vi "Teguh_2.vi"() -> ()   [LabVIEW 2024]
uses:
  <vilib>/Utility/NIReport.llb/Report Type.ctl
  <vilib>/MakerHub/LINX/Private/Device/Type Defs/Stimulus Pulse.ctl
  <vilib>/MakerHub/LINX/Public/Peripherals/Digital/Digital Write 1 Chan.vi
  <vilib>/MakerHub/LINX/Public/Peripherals/Digital/Digital Write N Chans.vi
  <vilib>/MakerHub/LINX/Private/Local IO/LinxDigitalWrite.vi
  <vilib>/MakerHub/LINX/Public/Utilities/Check Channel.vi
  <vilib>/MakerHub/LINX/Public/Utilities/Open Serial.vi
  <vilib>/MakerHub/LINX/Public/Sensors/Motion/Servo/Servo Open One Channel.vi
  <vilib>/Utility/NIReport.llb/Append Report Text (str wrap).vi
  <vilib>/Utility/NIReport.llb/Append Text Table to Report (wrap).vi
  <vilib>/MakerHub/LINX/Private/Utilties/Generate Error.vi
  <vilib>/MakerHub/LINX/Public/Sensors/Motion/Servo/Servo Set Pulse Width One Channel.vi
  <vilib>/MakerHub/LINX/Public/Sensors/Motion/Servo/Servo Close One Channel.vi
  <vilib>/Utility/NIReport.llb/NI_report.lvclass
  <vilib>/MakerHub/LINX/LMH-LINX.lvlib
  <vilib>/MakerHub/LINX/Public/Sensors/Motion/Servo/Servo.lvlib
  <vilib>/Analysis/NI_AALPro.lvlib
  <vilib>/MakerHub/LINX/Private/Device/Device.lvlib
  <vilib>/Utility/NIReport.llb/Excel/NI_Excel.lvclass
  <vilib>/Utility/NIReport.llb/NI_ReportGenerationCore.lvlib
panel:
  out "Jarak Dalam Centimeter":dbl(slide) scale=0.0..60.0
  in  "report file path 2":path
  out "output array":string[][](array[string])
  in  "Directory Excel":path
  out "Pulse Width (uS)":i32(slide) scale=0.0..4000.0
  in  "Trigg out":u8
  in  "Echo in":u8
  out "Time String":string
  out "Data String":string
  in  "SERVO TUTUP":dbl format="%0.2f"
  in  "Kurang Dari":dbl
  in  "SERIAL PORT":refnum<visa-resource-name>="N/A"
  in  "?":bool
  in  "SERVO BUKA":dbl format="%0.2f"
  # "PROGRAM TEMPAT SAMPAH OTOMATIS OTOMATIS"
  # "Tanggal"
  # "Waktu"
  # "Kondisi"
  # "Jarak"
  # "TEGUH KECE"
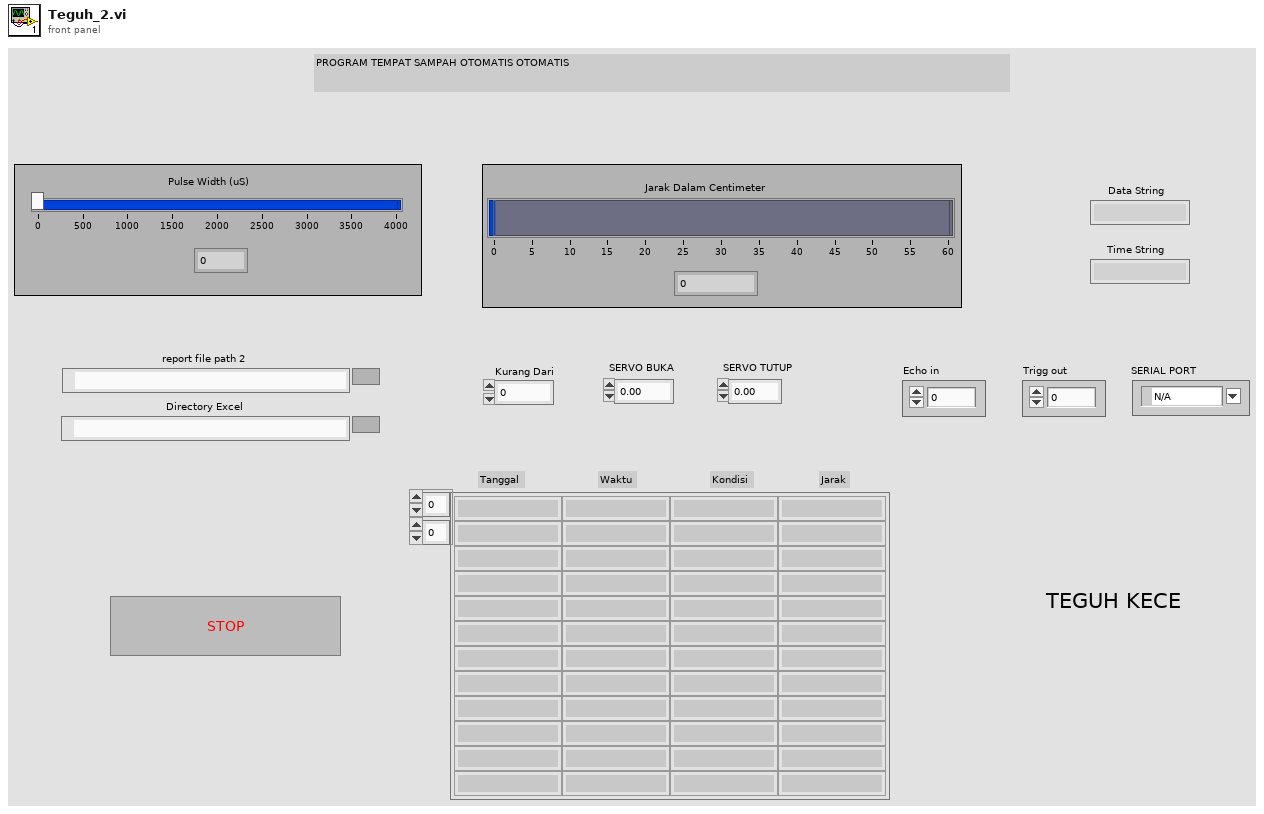
[diagram p1: front panel]
types:
  T1 = typedef "NI_ReportGenerationCore.lvlib/Report Type.ctl" = enum16{"HTML", "Word", "Excel"}
  T2 = typedef "LMH-LINX.lvlib/LINX Ref.ctl" = cluster{"IO":T3, "Interface":T4, "LINX Device Config":T5}
  T3 = typedef "LMH-LINX.lvlib/Platform.ctl" = enum16{"Remote", "Local"}
  T4 = typedef "LMH-LINX.lvlib/Interface.ctl" = enum16{"Serial", "TCP"}
  T5 = typedef "LMH-LINX.lvlib/Device.lvlib/LINX Device Config.ctl" = cluster{"Interface":T4, "COM Port":refnum<visa-resource-name>, "TCP Configuration":T6, "Device Family":u8, "Device ID":u8, "Device Name":string, "TCP Ref":refnum<k5>, "Channels":T7}
  T6 = typedef "LMH-LINX.lvlib/Device.lvlib/TCP Config.ctl" = cluster{"IP Address":string, "Port":u16}
  T7 = typedef "LMH-LINX.lvlib/Channels.ctl" = cluster{"DI":u8[], "DO":u8[], "AI":u8[], "AO":u8[], "PWM":u8[], "QE":u8[], "UART":u8[], "I2C 2":u8[], "SPI":u8[], "CAN":u8[], "Servo":u8[], "AI Ref (V)":dbl, "AI Resolution (Bits)":u8, "AO Ref (V)":dbl, "AO Resolution (Bits)":u8}
  T8 = typedef "LMH-LINX.lvlib/Device.lvlib/Stimulus Pulse.ctl" = enum16{"None", "Active Low", "Active High"}
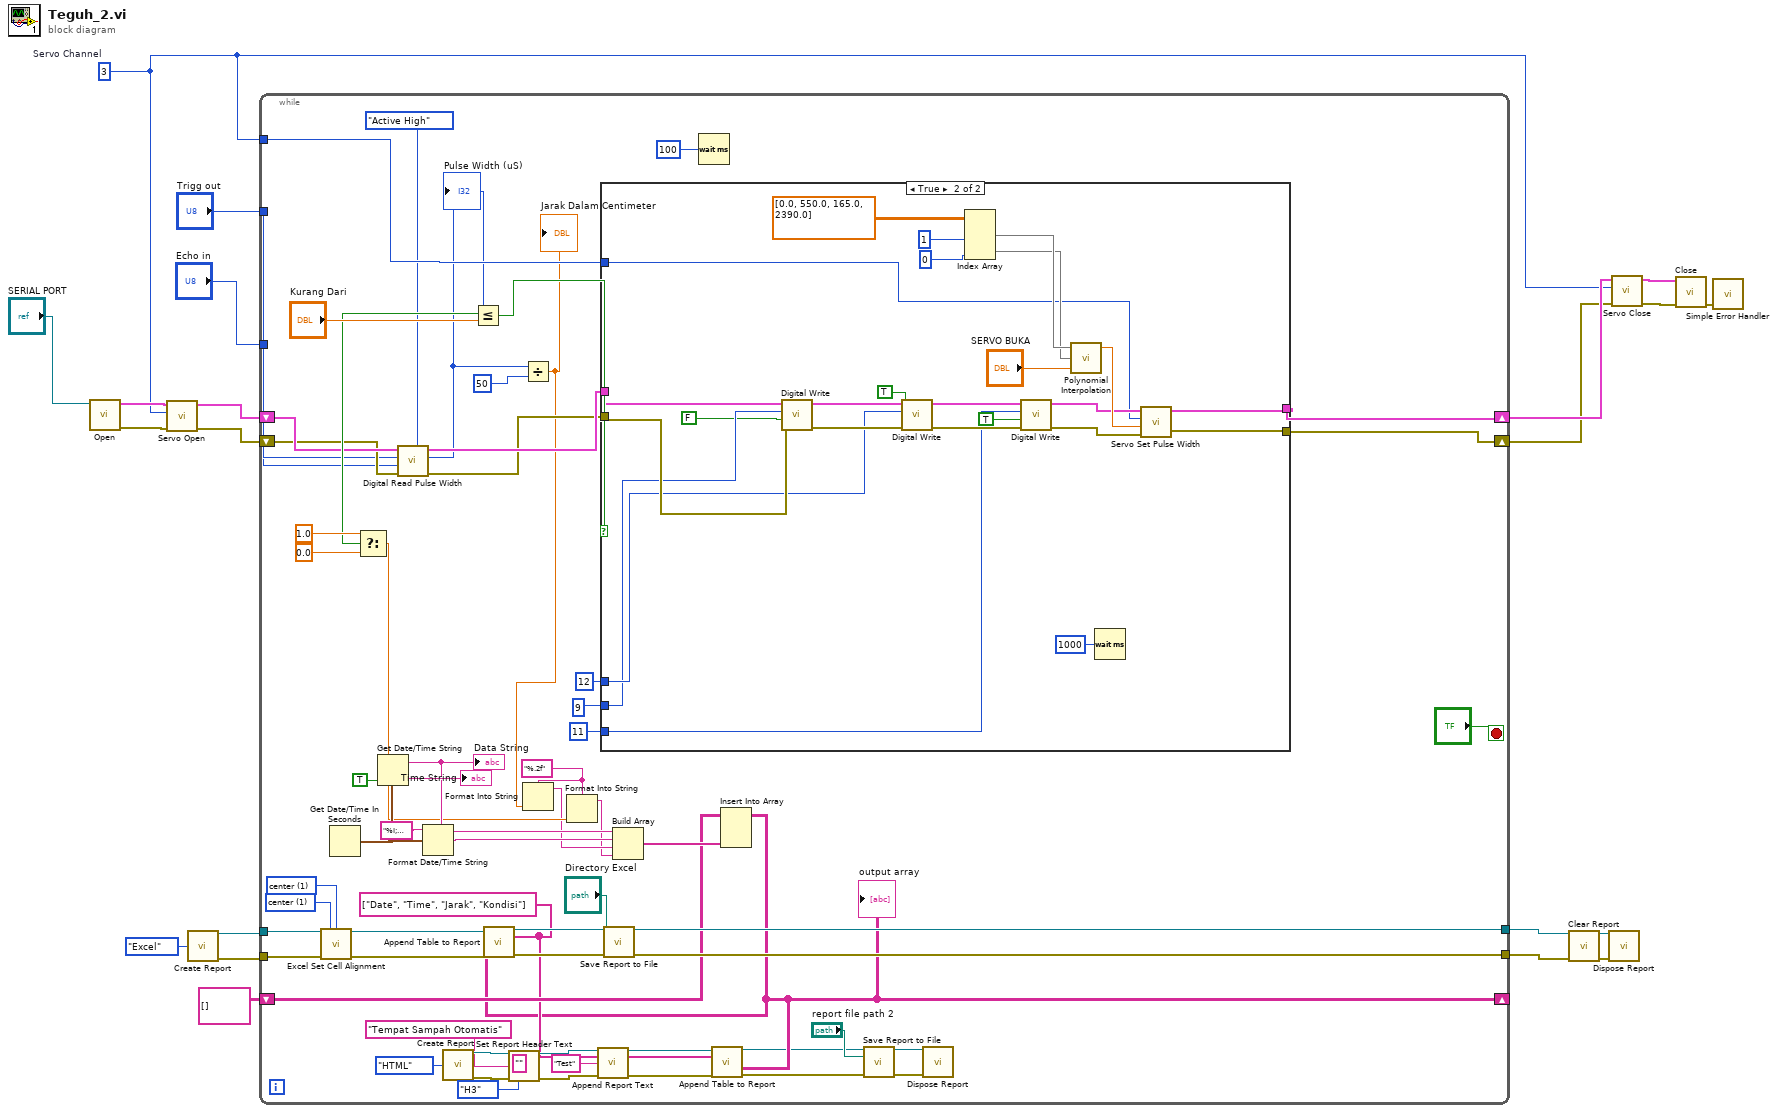
[diagram p0: block diagram]
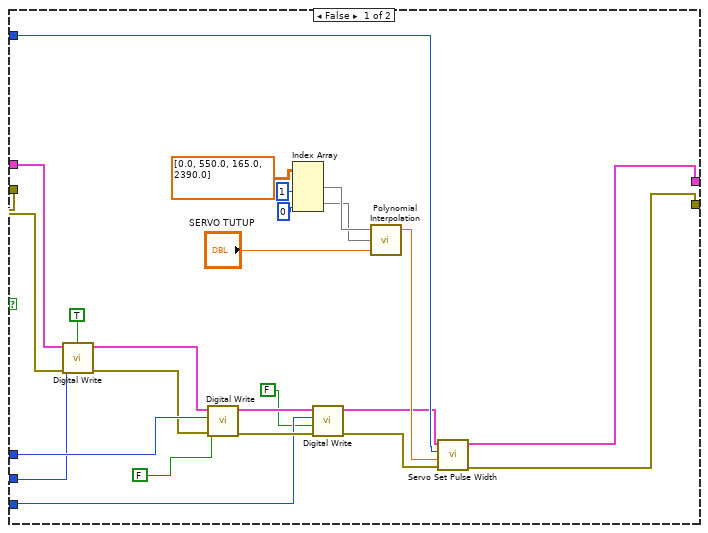
[diagram p2: hidden frame]
diagram:
  w11 = u8 3  # Servo Channel
  n1 = call-poly <vilib>:"Open.vi"("Serial Port"="SERIAL PORT") -> ("Error Out"=w19:errorcluster, "LINX Resource"=w21:T2)  [unwired: 8 in, 1 out]
  n2 = call-poly <vilib>:"Servo Open.vi"("Error In"=w19, "Servo Channel"=w11, "LINX Resource"=w21) -> ("Error Out"=w14:errorcluster, "LINX Resource"=w20:T2)  [unwired: 7 in]
  n3 = call <vilib>:"Create Report.vi"("report type"=Report_Type."Excel") -> ("report out"=w8:refnum<class "NI_report.lvclass">, "error out"=w7:errorcluster)  [unwired: 13 in]
  n4 = while {
    shift-right: [w78] -> w18
    shift-left: w20 -> [w67]
    shift-right: [w77] -> w16
    shift-left: w14 -> [w66]
    tunnel: w11 -> [w70]
    tunnel: "Echo in" -> [w64]
    tunnel: "Trigg out" -> [w63]
    tunnel: w8 -> [w62]
    tunnel: w7 -> [w61]
    tunnel: [w56] -> w6
    tunnel: [w55] -> w5
    shift-right: [w30] -> _
    shift-left: string[][] [] -> [w45]
    stop <- "?" stop-if-true
    (unwired) "" ("text")
    w43 = "%.2f" ("format string")
    w31 = string[] ["Date", "Time", "Jarak", "Kondisi"] ("column headers")
    w53 = 1 items=["left", "center", "right"] ("horizontal alignment (left)")
    w54 = 1 items=["top", "center", "bottom"] ("vertical alignment (top)")
    n5 = call <vilib>:"Excel Set Cell Alignment.vi"("report in"=w62, "vertical alignment (top)"=w54, "horizontal alignment (left)"=w53, "error in (no error)"=w61) -> ("report out"=w60:refnum<class "NI_report.lvclass">, "error out"=w59:errorcluster)  [unwired: 10 in]
    n6 = Get Date/Time In Seconds() -> (seconds since 1Jan1904=w52:timestamp)
    n7 = Get Date/Time String(seconds (now)=w52, want seconds? (F)=TRUE) -> (date string=w50:string, time string=→"Time String":string)  [unwired: 1 in]
    "Data String" <- w50
    n8 = call <vilib>:"Digital Read Pulse Width.vi"("Stimulus Pulse (Active High)"=Stimulus_Pulse."Active High", "Error In"=w66, "DO Channel"=w63, "DI Channel"=w64, "LINX Resource"=w67) -> ("Error Out"=w65:errorcluster, "Pulse Width (uS)"=w40:u32, "LINX Resource"=w68:T2)  [unwired: 4 in]
    "Pulse Width (uS)" <- w40
    n9 = Format Date/Time String(time format string (%c)="%I; %M; %S; %p", seconds (now)=w52) -> (date/time string=w49:string)  [unwired: 1 in]
    n10 = call <vilib>:"Create Report.vi"("report type"=Report_Type."HTML") -> ("report out"=w37:refnum<class "NI_report.lvclass">, "error out"=w36:errorcluster)  [unwired: 13 in]
    n11 = Less Or Equal?(x=w40, y="Kurang Dari") -> (x <= y?=w73:bool)
    n12 = Select(t=1.0, s=w73, f=0.0) -> (s? t:f=w47:dbl)
    n13 = call-dynamic "Set Report Header Text.vi"("report in"=w37, "center header text"="Tempat Sampah Otomatis", "error in (no error)"=w36, "HTML header size"=enum16{"H1", "H2", "H3", "H4", "H5", "H6", "H7"}."H3") -> ("report out"=w33:refnum<class "NI_report.lvclass">, "error out"=w32:errorcluster)  [unwired: 10 in]
    n14 = Divide(x=w40, y=u32 50) -> (x/y=w22:dbl)
    "Jarak Dalam Centimeter" <- w22
    n15 = Format Into String(format string=w43, w22) -> (resulting string=w42:string)  [unwired: 2 in, 1 out]
    n16 = Format Into String(format string=w43, w47) -> (resulting string=w41:string)  [unwired: 2 in, 1 out]
    n17 = call-poly <vilib>:"Append Report Text.vi"("report in"=w33, "text"="Test", "error in (no error)"=w32) -> ("report out"=w28:refnum<class "NI_report.lvclass">, "error out"=w27:errorcluster)  [unwired: 9 in, 2 out]
    n18 = case shown="True" w73 {
      tunnel: w68 -> [w96 w123]
      tunnel: w65 -> [w98 w122]
      tunnel: 12 ("code") -> [w100 w121]
      tunnel: 9 -> [w99 w120]
      tunnel: [w94 w119] -> w78
      tunnel: [w93 w118] -> w77
      tunnel: u8 11 ("DO Channel") -> [w87 w113]
      tunnel: w70 -> [w92 w112]
      frame False {
        n19 = call-poly <vilib>:"Digital Write.vi"("Error In"=w98, "Output Value"=TRUE, "DO Channel"=w99, "LINX Resource"=w96) -> ("Error Out"=w97:errorcluster, "LINX Resource"=w95:T2)  [unwired: 6 in]
        n20 = call-poly <vilib>:"Digital Write.vi"("Error In"=w97, "Output Value"=FALSE, "DO Channel"=w100, "LINX Resource"=w95) -> ("Error Out"=w90:errorcluster, "LINX Resource"=w91:T2)  [unwired: 6 in]
        n21 = Index Array(array=dbl[][] [[0.0, 550.0], [165.0, 2390.0]], index (col) #1=1 ("disabled index (col)"), index (col) #2=0 ("index (col)")) -> (element #1=w105:dbl[], element #2=w104:dbl[])  [unwired: 2 in]
        n22 = call-poly <vilib>:"Digital Write.vi"("Error In"=w90, "Output Value"=FALSE, "DO Channel"=w87, "LINX Resource"=w91) -> ("Error Out"=w88:errorcluster, "LINX Resource"=w89:T2)  [unwired: 6 in]
        n23 = call <vilib>:"Polynomial Interpolation.vi"("x value"="SERVO TUTUP", "X"=w104, "Y"=w105) -> ("interpolation value"=w107:dbl)  [unwired: 2 out]
        n24 = call-poly <vilib>:"Servo Set Pulse Width.vi"("Error In"=w88, "Pulse Width (uS)"=w107, "Servo Channel"=w92, "LINX Resource"=w89) -> ("Error Out"=w93:errorcluster, "LINX Resource"=w94:T2)  [unwired: 6 in]
      }
      frame True {
        n25 = call-poly <vilib>:"Digital Write.vi"("Error In"=w122, "Output Value"=FALSE, "DO Channel"=w120, "LINX Resource"=w123) -> ("Error Out"=w125:errorcluster, "LINX Resource"=w124:T2)  [unwired: 6 in]
        n26 = call-poly <vilib>:"Digital Write.vi"("Error In"=w125, "Output Value"=TRUE, "DO Channel"=w121, "LINX Resource"=w124) -> ("Error Out"=w115:errorcluster, "LINX Resource"=w117:T2)  [unwired: 6 in]
        n27 = Index Array(array=dbl[][] [[0.0, 550.0], [165.0, 2390.0]], index (col) #1=1 ("disabled index (col)"), index (col) #2=0 ("index (col)")) -> (element #1=w130:dbl[], element #2=w129:dbl[])  [unwired: 2 in]
        n28 = call-poly <vilib>:"Digital Write.vi"("Error In"=w115, "Output Value"=TRUE, "DO Channel"=w113, "LINX Resource"=w117) -> ("Error Out"=w114:errorcluster, "LINX Resource"=w116:T2)  [unwired: 6 in]
        n29 = call <vilib>:"Polynomial Interpolation.vi"("x value"="SERVO BUKA", "X"=w129, "Y"=w130) -> ("interpolation value"=w132:dbl)  [unwired: 2 out]
        n30 = Wait (ms)(milliseconds to wait=u32 1000) -> ()  [unwired: 1 out]
        n31 = call-poly <vilib>:"Servo Set Pulse Width.vi"("Error In"=w114, "Pulse Width (uS)"=w132, "Servo Channel"=w112, "LINX Resource"=w116) -> ("Error Out"=w118:errorcluster, "LINX Resource"=w119:T2)  [unwired: 6 in]
      }
    }
    n32 = Build Array(w50, w49, w42, w41) -> (w46:string[])
    n33 = Wait (ms)(milliseconds to wait=u32 100) -> ()  [unwired: 1 out]
    n34 = Insert Into Array(array=w45, new element=w46) -> (w30:string[][])  [unwired: 2 in]
    "output array" <- w30
    n35 = call-poly <vilib>:"Append Table to Report.vi"("report in"=w60, "column headers"=w31, "text data"=w30, "error in (no error)"=w59) -> ("report out"=w58:refnum<class "NI_report.lvclass">, "error out"=w57:errorcluster)  [unwired: 8 in, 2 out]
    n36 = call-dynamic "Save Report to File.vi"("report in"=w58, "report file path"="Directory Excel", "error in (no error)"=w57) -> ("report out"=w56:refnum<class "NI_report.lvclass">, "error out"=w55:errorcluster)  [unwired: 11 in]
    n37 = call-poly <vilib>:"Append Table to Report.vi"("report in"=w28, "column headers"=w31, "text data"=w30, "error in (no error)"=w27) -> ("report out"=w26:refnum<class "NI_report.lvclass">, "error out"=w25:errorcluster)  [unwired: 8 in, 2 out]
    n38 = call-dynamic "Save Report to File.vi"("report in"=w26, "report file path"="report file path 2", "error in (no error)"=w25) -> ("report out"=w24:refnum<class "NI_report.lvclass">, "error out"=w23:errorcluster)  [unwired: 11 in]
    n39 = call-dynamic "Dispose Report.vi"("report in"=w24, "error in (no error)"=w23) -> ()  [unwired: 13 in, 1 out]
  }
  n40 = call-dynamic "Clear Report.vi"("report in"=w6, "error in (no error)"=w5) -> ("report out"=w4:refnum<class "NI_report.lvclass">, "error out"=w3:errorcluster)  [unwired: 12 in]
  n41 = call-dynamic "Dispose Report.vi"("report in"=w4, "error in (no error)"=w3) -> ()  [unwired: 13 in, 1 out]
  n42 = call-poly <vilib>:"Servo Close.vi"("Error In"=w16, "Servo Channel"=w11, "LINX Resource"=w18) -> ("Error Out"=w15:errorcluster, "LINX Resource"=w17:T2)  [unwired: 7 in]
  n43 = call <vilib>:"Close.vi"("Error In"=w15, "LINX Resource"=w17) -> ("Error Out"=w13:errorcluster)  [unwired: 9 in]
  n44 = call <vilib>:"Simple Error Handler.vi"("error in (no error)"=w13) -> ()  [unwired: 4 in, 5 out]
